vi "JSON_Si_Parser (SubVI).vi"(6 "data":string, 8 "error in (no error)":errorcluster, 9 "Numeric":i32) -> (0 "error out":errorcluster, 2 "Cluster":T1)   [LabVIEW 2018]
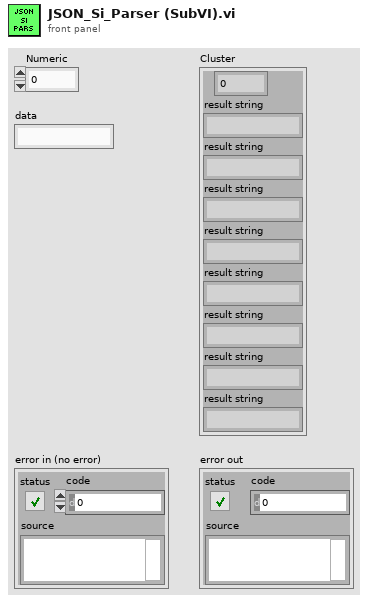
[diagram p1: front panel]
types:
  T1 = cluster{i32, "result string":string, "result string":string, "result string":string, "result string":string, "result string":string, "result string":string, "result string":string, "result string":string}
  T2 = cluster{"Numeric":i32, "result string":string, "result string":string, "result string":string, "result string":string, "result string":string, "result string":string, "result string":string, "result string":string}
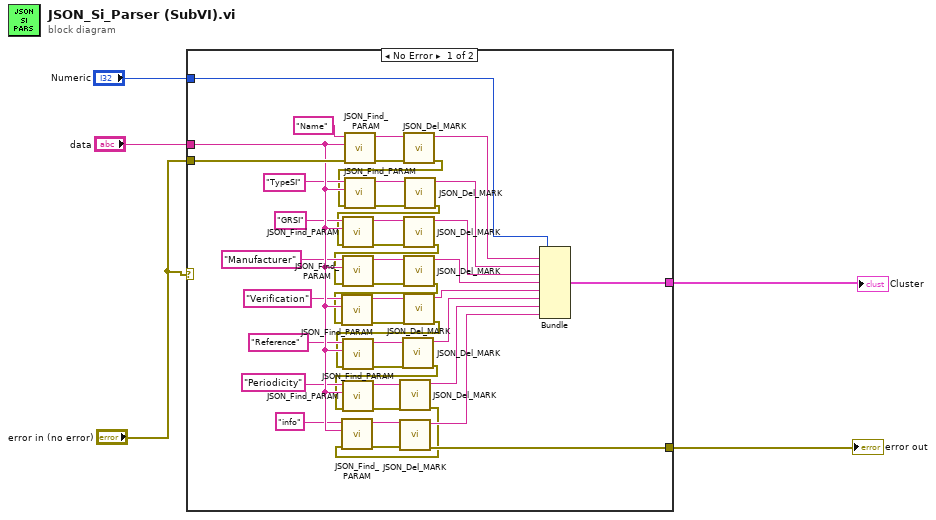
[diagram p0: block diagram]
diagram:
  n1 = case shown="No Error" "error in (no error)" {
    tunnel: [w49 w50] -> w5
    tunnel: "error in (no error)" -> [w48 w50]
    tunnel: "data" -> [w23 _]
    tunnel: "Numeric" -> [w6 _]
    tunnel: [w14 _] -> w2
    frame No Error {
      n2 = call "JSON_Find_PARAM.vi"("error in (no error)"=w48, "data"=w23, "name"="Name") -> ("error out"=w24:errorcluster, "String"=w25:string)  [unwired: 7 in]
      n3 = call "JSON_Del_MARK.vi"("error in (no error)"=w24, "String"=w25) -> ("error out"=w13:errorcluster, "result string"=w40:string)  [unwired: 8 in]
      n4 = call "JSON_Find_PARAM.vi"("error in (no error)"=w13, "data"=w23, "name"="TypeSI") -> ("error out"=w27:errorcluster, "String"=w26:string)  [unwired: 7 in]
      n5 = call "JSON_Del_MARK.vi"("error in (no error)"=w27, "String"=w26) -> ("error out"=w12:errorcluster, "result string"=w41:string)  [unwired: 8 in]
      n6 = call "JSON_Find_PARAM.vi"("error in (no error)"=w12, "data"=w23, "name"="GRSI") -> ("error out"=w29:errorcluster, "String"=w28:string)  [unwired: 7 in]
      n7 = call "JSON_Del_MARK.vi"("error in (no error)"=w29, "String"=w28) -> ("error out"=w11:errorcluster, "result string"=w42:string)  [unwired: 8 in]
      n8 = call "JSON_Find_PARAM.vi"("error in (no error)"=w11, "data"=w23, "name"="Manufacturer") -> ("error out"=w31:errorcluster, "String"=w30:string)  [unwired: 7 in]
      n9 = call "JSON_Del_MARK.vi"("error in (no error)"=w31, "String"=w30) -> ("error out"=w10:errorcluster, "result string"=w43:string)  [unwired: 8 in]
      n10 = call "JSON_Find_PARAM.vi"("error in (no error)"=w10, "data"=w23, "name"="Verification") -> ("error out"=w33:errorcluster, "String"=w32:string)  [unwired: 7 in]
      n11 = call "JSON_Del_MARK.vi"("error in (no error)"=w33, "String"=w32) -> ("error out"=w9:errorcluster, "result string"=w44:string)  [unwired: 8 in]
      n12 = call "JSON_Find_PARAM.vi"("error in (no error)"=w9, "data"=w23, "name"="Reference") -> ("error out"=w35:errorcluster, "String"=w34:string)  [unwired: 7 in]
      n13 = call "JSON_Del_MARK.vi"("error in (no error)"=w35, "String"=w34) -> ("error out"=w8:errorcluster, "result string"=w45:string)  [unwired: 8 in]
      n14 = call "JSON_Find_PARAM.vi"("error in (no error)"=w8, "data"=w23, "name"="Periodicity") -> ("error out"=w37:errorcluster, "String"=w36:string)  [unwired: 7 in]
      n15 = call "JSON_Del_MARK.vi"("error in (no error)"=w37, "String"=w36) -> ("error out"=w7:errorcluster, "result string"=w46:string)  [unwired: 8 in]
      n16 = call "JSON_Find_PARAM.vi"("error in (no error)"=w7, "data"=w23, "name"="info") -> ("error out"=w39:errorcluster, "String"=w38:string)  [unwired: 7 in]
      n17 = call "JSON_Del_MARK.vi"("error in (no error)"=w39, "String"=w38) -> ("error out"=w49:errorcluster, "result string"=w47:string)  [unwired: 8 in]
      n18 = Bundle("Numeric"=w6, "result string"=w40, "result string"=w41, "result string"=w42, "result string"=w43, "result string"=w44, "result string"=w45, "result string"=w46, "result string"=w47) -> (w14:T2)  [unwired: 1 in]
    }
    frame Error {
    }
  }
  "error out" <- w5
  "Cluster" <- w2
